vi "Check Null Pointer.vi"(7 "source vi name":string, 8 "error in (no error)":errorcluster, 11 "Pointer in":refnum<class "Pointer.lvclass">) -> (0 "error out":errorcluster, 3 "Pointer out":refnum<class "Pointer.lvclass">)   [LabVIEW 2017, in "Memory Manager.lvlib" / "Pointer.lvclass"]
uses:
  Pointer.lvclass
  Error VIs/Null Pointer.vi
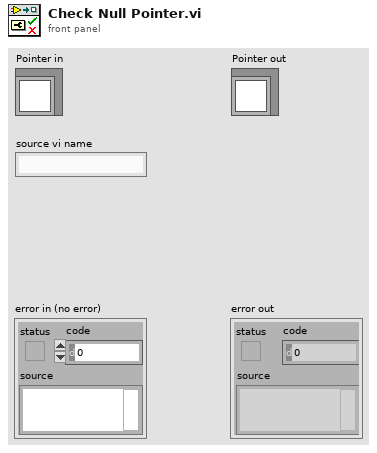
[diagram p1: front panel]
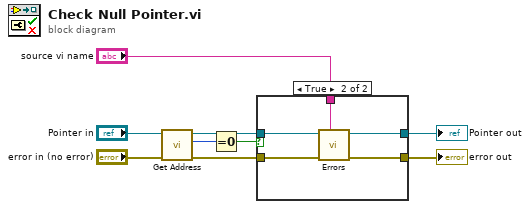
[diagram p0: block diagram]
diagram:
  n1 = call "Get Address.vi"("Pointer in"="Pointer in") -> ("address"=w6:u64, "Pointer out"=w3:refnum<class "Pointer.lvclass">)  [unwired: 9 in]
  n2 = Equal To 0?(x=w6) -> (x = 0?=w4:bool)
  n3 = case shown="True" w4 {
    tunnel: w3 -> [w9 w15]
    tunnel: "error in (no error)" -> [w10 w13]
    tunnel: [w10 w12] -> w8
    tunnel: [w9 w14] -> w7
    tunnel: "source vi name" -> [_ w11]
    frame False {
    }
    frame True {
      n4 = call-poly "Errors.vi"("error source vi name"=w11, "error in (no error)"=w13, "Pointer in"=w15) -> ("error out"=w12:errorcluster, "Pointer out"=w14:refnum<class "Pointer.lvclass">)  [unwired: 7 in]
    }
  }
  "error out" <- w8
  "Pointer out" <- w7
